vi "Generate Overlap SQL Query.vi"(8 "error in (no error)":errorcluster, 11 "Importing Transactions":refnum<class "Statement.lvclass">) -> (0 "error out":errorcluster, 2 "Overlap Query":string, 3 "Overlapping Records":refnum<class "Statement.lvclass">)   [LabVIEW 2018, in "Statement.lvclass"]
uses:
  Statement.lvclass
  Statement.lvclass/Statement.ctl
  Transaction/Transaction.lvclass
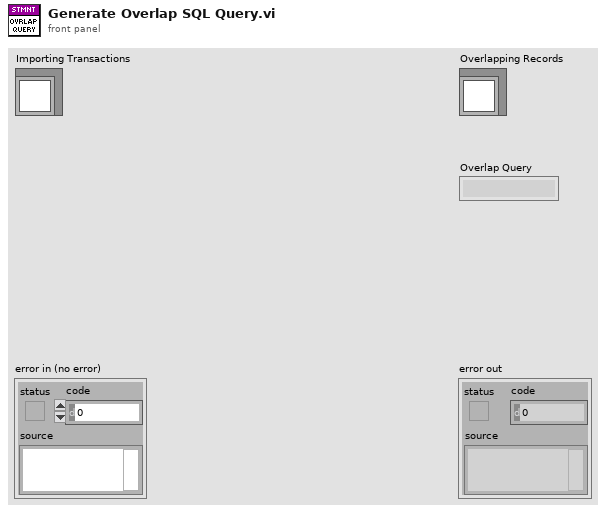
[diagram p1: front panel]
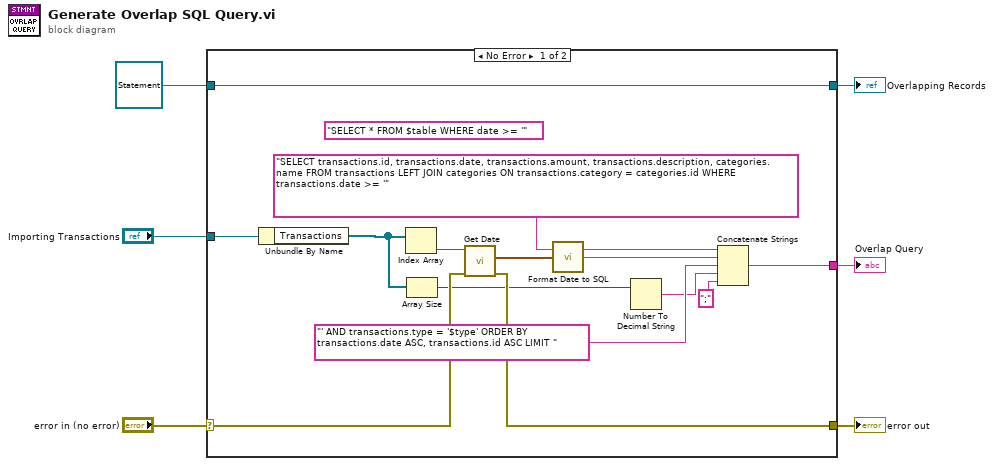
[diagram p0: block diagram]
diagram:
  n1 = case shown="No Error" "error in (no error)" {
    selector: "error in (no error)" -> [w12 w22]
    tunnel: [w11 w22] -> w5
    tunnel: "Importing Transactions" -> [w16 _]
    tunnel: [w10 _] -> w3
    tunnel: refnum<class "Statement.lvclass"> refnum ("Statement.lvclass") -> [w8 w21]
    tunnel: [w8 w21] -> w1
    frame No Error {
      (unwired) "SELECT * FROM $table WHERE date >= '"
      n2 = Unbundle By Name(w16) -> ("Transactions"=w15:refnum<class "Transaction.lvclass">[])
      n3 = Index Array(array=w15) -> (element=w14:refnum<class "Transaction.lvclass">)  [unwired: 1 in]
      n4 = Array Size(array=w15) -> (size(s)=w9:i32)
      n5 = call "Get Date.vi"("error in (no error)"=w12, "Transaction in"=w14) -> ("error out"=w11:errorcluster, "Date"=w13:timestamp)  [unwired: 7 in, 1 out]
      n6 = call "Format Date to SQL.vi"("Date"=w13) -> ("SQL Date"=w17:string)
      n7 = Number To Decimal String(number=w9) -> (decimal integer string=w19:string)  [unwired: 1 in]
      n8 = Concatenate Strings("SELECT transactions.id, transactions.date, transactions.amount, transactions.description, categories.name FROM transactions LEFT JOIN categories ON transactions.category = categories.id WHERE transactions.date >= '", w17, "' AND transactions.type = '$type' ORDER BY transactions.date ASC, transactions.id ASC LIMIT " ("string"), w19, ";" ("string")) -> (w10:string)
    }
    frame Error {
    }
  }
  "error out" <- w5
  "Overlapping Records" <- w1
  "Overlap Query" <- w3
